vi "CRYPlot Curve Library.vi"(6 "Waveform":T2[](array[typedef]) {"Y dB ref" format="%.1f"; "Y axis" items=["Log", "Lin"]; "Y data" items=["dB", "Lin"]; "X data" items=["dB", "Lin"]}, 8 "Results":T3[](array[typedef]) {"Margin" format="%.2f"}, 9 "Values":T1[](array[typedef]) {"Z data" items=["dB", "Lin"]; "X data" items=["dB", "Lin"]; "Y data" items=["dB", "Lin"]; "Z dB ref" format="%.1f"; "Z axis" items=["Log", "Lin"]; "X dB ref" format="%.1f"; "X axis" items=["Log", "Lin"]; "Y axis" items=["Log", "Lin"]; "Y dB ref" format="%.1f"; "Curve"."z" format="%.2f"; "Curve"."y" format="%.2f"; "Curve"."x" format="%.2f"}, 10 "Curves":T1[](array[typedef]) {"Z data" items=["dB", "Lin"]; "X data" items=["dB", "Lin"]; "Y data" items=["dB", "Lin"]; "Z dB ref" format="%.1f"; "Z axis" items=["Log", "Lin"]; "X dB ref" format="%.1f"; "X axis" items=["Log", "Lin"]; "Y axis" items=["Log", "Lin"]; "Y dB ref" format="%.1f"; "Curve"."z" format="%.2f"; "Curve"."y" format="%.2f"; "Curve"."x" format="%.2f"}, 11 "Type":enum16{"Curves", "Values", "Results", "WFM"}(ring)) -> (3 "PlotStrings":string[][](array[string]))   [LabVIEW 2013]
uses:
  CRYSystem/Typedef Control/CRYData Cluster.ctl
  CRYSystem/Typedef Control/CRYResult Cluster.ctl
  CRYSystem/Typedef Control/CRYWaveform Cluster.ctl
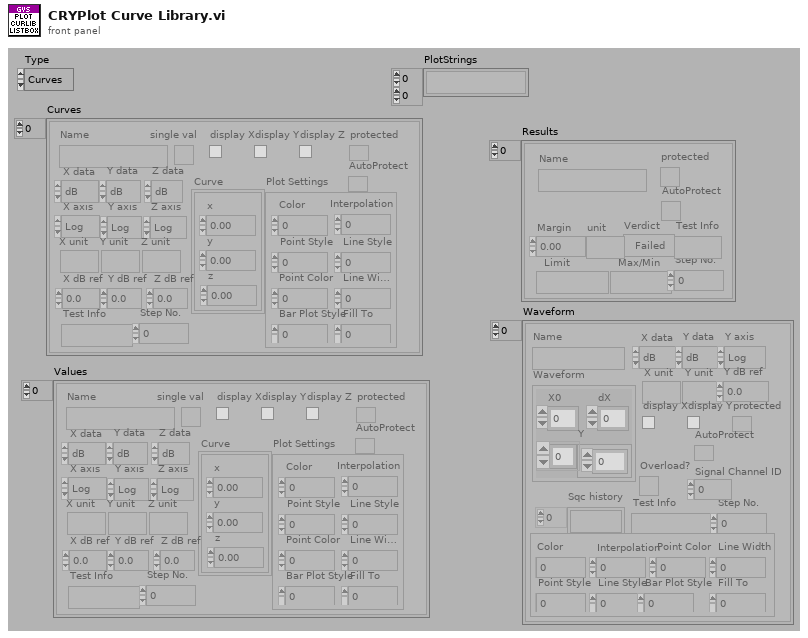
[diagram p1: front panel]
types:
  T1 = typedef "CRYData Cluster.ctl" = cluster{"Name":string, "Curve":cluster{"x":dbl, "y":dbl, "z":dbl}[], "X data":u16, "Y data":u16, "Z data":u16, "X axis":u16, "Y axis":u16, "Z axis":u16, "X unit":string, "Y unit":string, "Z unit":string, "X dB ref":dbl, "Y dB ref":dbl, "Z dB ref":dbl, "single val":bool, "protected":bool, "display X":bool, "display Y":bool, "display Z":bool, "Test Info":string, "Step No.":i32, "Plot Settings":cluster{"Color":u32, "Interpolation":u8, "Point Style":u8, "Line Style":u8, "Point Color":u32, "Line Width":u8, "Bar Plot Style":u8, "Fill To":i16}, "AutoProtect":bool}
  T2 = typedef "CRYWaveform Cluster.ctl" = cluster{"Waveform":cluster{"X0":dbl, "dX":dbl, "Y":sgl[]}, "X data":u16, "Y data":u16, "Y axis":u16, "X unit":string, "Y unit":string, "Y dB ref":dbl, "display Y":bool, "display X":bool, "Overload?":bool, "Test Info":string, "Step No.":i32, "Name":string, "protected":bool, "Sqc history":string[], "Signal Channel ID":i32, "Plot Settings":cluster{"Color":u32, "Interpolation":u8, "Point Style":u8, "Line Style":u8, "Point Color":u32, "Line Width":u8, "Bar Plot Style":u8, "Fill To":i16}, "AutoProtect":bool}
  T3 = typedef "CRYResult Cluster.ctl" = cluster{"Name":string, "Margin":dbl, "unit":string, "Verdict":bool, "Limit":string, "Max/Min":string, "protected":bool, "Step No.":i32, "Test Info":string, "AutoProtect":bool}
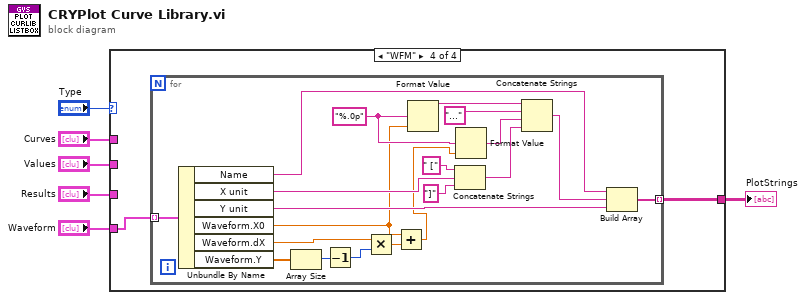
[diagram p0: block diagram]
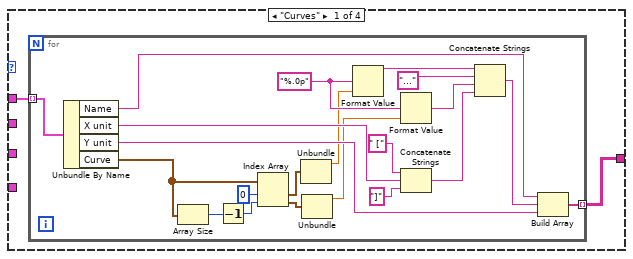
[diagram p2: hidden frame]
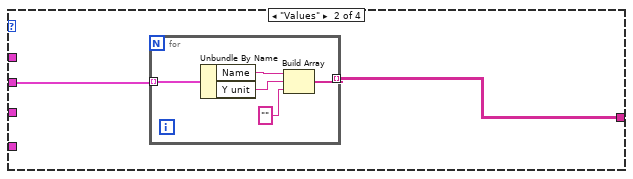
[diagram p3: hidden frame]
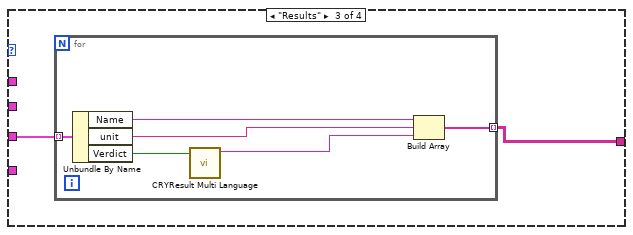
[diagram p4: hidden frame]
diagram:
  n1 = case shown="\"WFM\"" "Type" {
    tunnel: [w8 w31 w38 w46] -> w2
    tunnel: "Curves" -> [w7 _ _ _]
    tunnel: "Results" -> [_ _ w37 _]
    tunnel: "Waveform" -> [_ _ _ w45]
    tunnel: "Values" -> [_ w30 _ _]
    frame "Curves" {
      n2 = for {
        tunnel: w7 -> [w12] mode=indexing
        tunnel: [w11] -> w8 mode=indexing
        w20 = "%.0p" ("format string")
        n3 = Unbundle By Name(w12) -> ("Name"=w10:string, "X unit"=w21:string, "Y unit"=w25:string, "Curve"=w19:cluster{"x":dbl, "y":dbl, "z":dbl}[])
        n4 = Array Size(array=w19) -> (size(s)=w9:i32)
        n5 = Decrement(x=w9) -> (x-1=w17:i32)
        n6 = Index Array(array=w19, index #1=0 ("index"), index #2=w17) -> (element #1=w16:cluster{"x":dbl, "y":dbl, "z":dbl}, element #2=w15:cluster{"x":dbl, "y":dbl, "z":dbl})
        n7 = Unbundle(w16) -> ("x"=w13:dbl)  [unwired: 2 out]
        n8 = Unbundle(w15) -> ("x"=w14:dbl)  [unwired: 2 out]
        n9 = Format Value(format string=w20, value (0)=w13) -> (output string=w27:string)  [unwired: 1 in]
        n10 = Format Value(format string=w20, value (0)=w14) -> (output string=w29:string)  [unwired: 1 in]
        n11 = Concatenate Strings(" [", w21, "]") -> (w22:string)
        n12 = Concatenate Strings(w27, "...", w29, w22) -> (w26:string)
        n13 = Build Array(w10, w26, w25) -> (w11:string[])
      }
    }
    frame "Values" {
      n14 = for {
        tunnel: w30 -> [w35] mode=indexing
        tunnel: [w34] -> w31 mode=indexing
        n15 = Unbundle By Name(w35) -> ("Name"=w33:string, "Y unit"=w36:string)
        n16 = Build Array(w33, w36, "" ("element")) -> (w34:string[])
      }
    }
    frame "Results" {
      n17 = for {
        tunnel: w37 -> [w43] mode=indexing
        tunnel: [w42] -> w38 mode=indexing
        n18 = Unbundle By Name(w43) -> ("Name"=w41:string, "unit"=w44:string, "Verdict"=w40:bool)
        n19 = call "CRYResult Multi Language.vi"("Verdict"=w40) -> ("ASCII out"=w39:string)  [unwired: 10 in]
        n20 = Build Array(w41, w44, w39) -> (w42:string[])
      }
    }
    frame "WFM" {
      n21 = for {
        tunnel: w45 -> [w53] mode=indexing
        tunnel: [w52] -> w46 mode=indexing
        w66 = "%.0p" ("format string")
        n22 = Unbundle By Name(w53) -> ("Name"=w51:string, "X unit"=w63:string, "Y unit"=w65:string, "Waveform.X0"=w50:dbl, "Waveform.dX"=w60:dbl, "Waveform.Y"=w58:sgl[])
        n23 = Array Size(array=w58) -> (size(s)=w59:i32)
        n24 = Decrement(x=w59) -> (x-1=w47:i32)
        n25 = Multiply(x=w60, y=w47) -> (x*y=w49:dbl)
        n26 = Add(x=w50, y=w49) -> (x+y=w48:dbl)
        n27 = Format Value(format string=w66, value (0)=w50) -> (output string=w54:string)  [unwired: 1 in]
        n28 = Concatenate Strings(" [", w63, "]") -> (w64:string)
        n29 = Format Value(format string=w66, value (0)=w48) -> (output string=w56:string)  [unwired: 1 in]
        n30 = Concatenate Strings(w54, "...", w56, w64) -> (w57:string)
        n31 = Build Array(w51, w57, w65) -> (w52:string[])
      }
    }
  }
  "PlotStrings" <- w2
